vi "Humid Air Total Transfered Energy Calculator & OutPut Tempratures.vi"(2 "MFRHA\nMass Flow Rate of Humid Air (Kg/s)":dbl[unit], 3 "Gas Presure":dbl[unit]=80000.0 min=80000.0 max=120000.0, 4 "T_AU":dbl[unit], 5 "Tceg":dbl[unit], 6 "RH Heat Exchanger Quality":dbl, 7 "RH":dbl) -> (0 "Mass Flow Rate of Humid Air of Out Put":dbl[unit], 1 "ToTal Transferd Energy of Air":dbl[unit])   [LabVIEW 2018]
panel:
  out "T_AU\nEvaporator Hot and Humaid Outlet \nAir Temprature":dbl[unit](slide) scale=0.0..100.0
  out "ToTal Transferd Energy of Air":dbl[unit](slide) scale=0.0..5000.0
  out "Humidity of Input Air":dbl(knob) scale=0.0..100.0
  out "Temprature Of Input Air\nKelvin Degree":dbl[unit](slide) scale=273.0..373.0
  out "Tk":dbl[unit]
  out "Temprature Of Input Air\nCentigrade Degree":dbl[unit](slide) scale=0.0..100.0
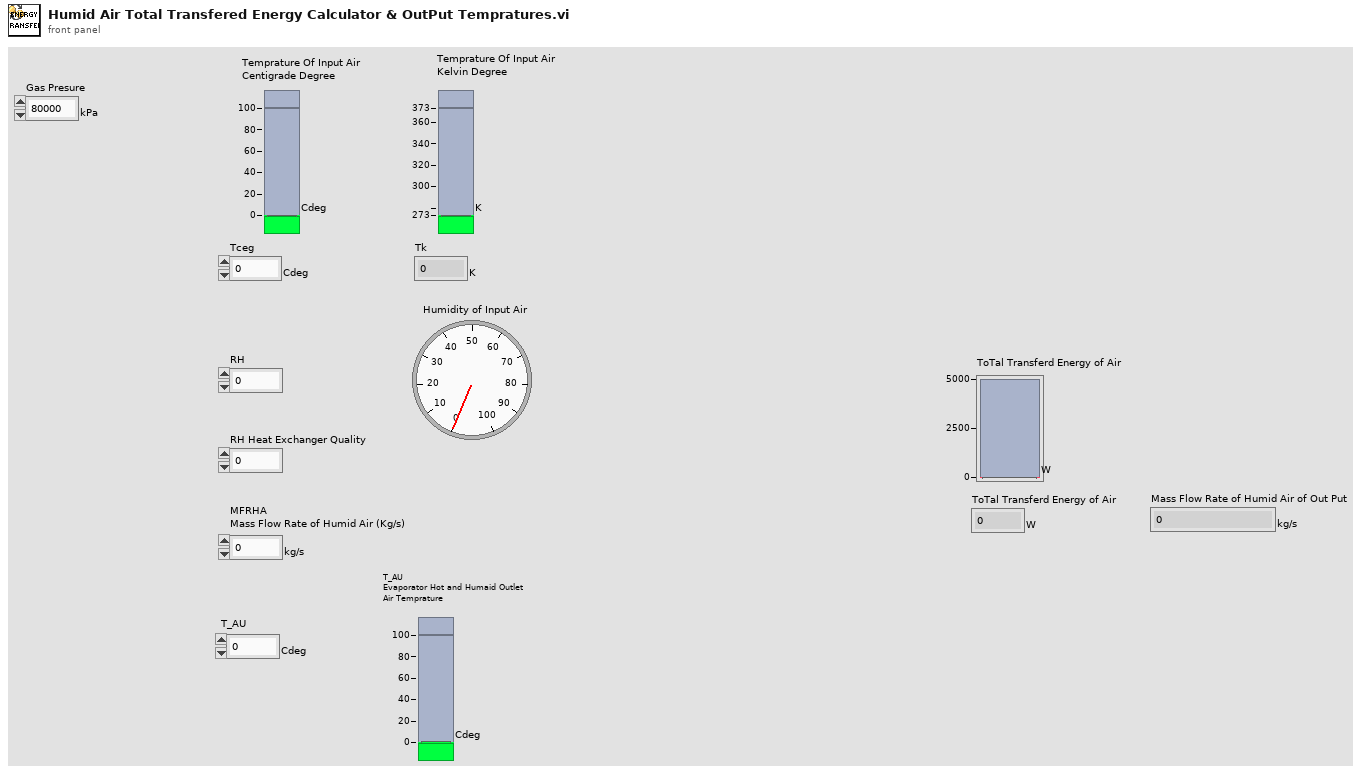
[diagram p1: front panel]
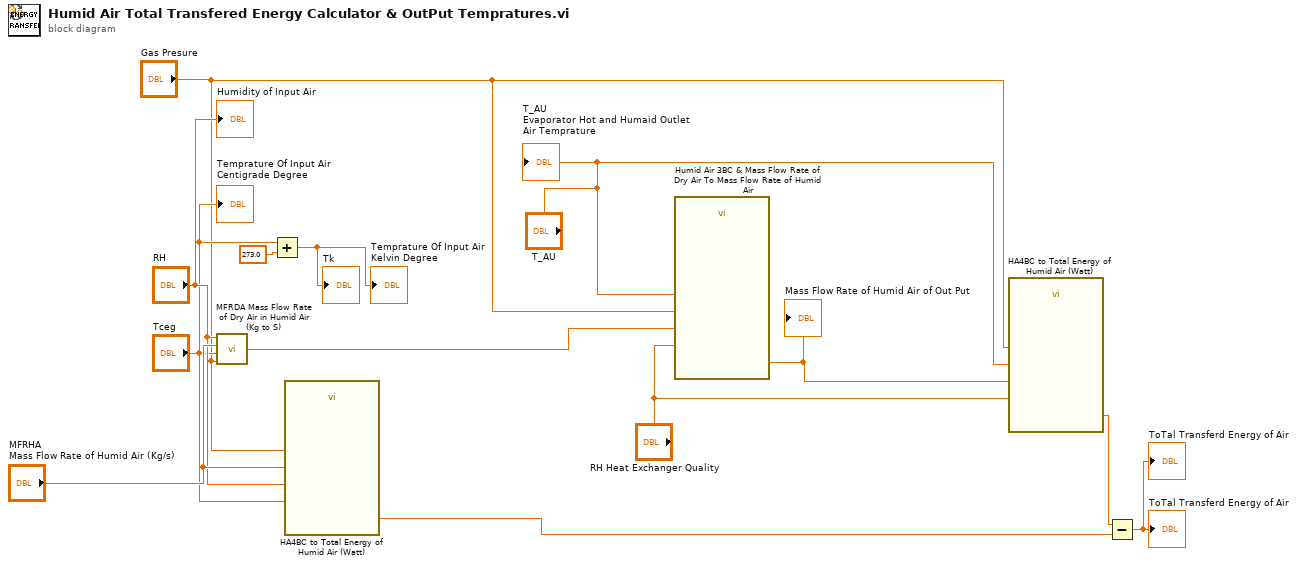
[diagram p0: block diagram]
diagram:
  n1 = call "MFRDA Mass Flow Rate of Dry Air in Humid Air (Kg to S).vi"("Gas Presure"="Gas Presure", "Tceg"="Tceg", "MFRHA\nMass Flow Rate of Humid Air (Kg/s)"="MFRHA\nMass Flow Rate of Humid Air (Kg/s)", "RH"="RH") -> ("MFRDA"=w11:dbl[unit])
  n2 = Add(x="Tceg", y=dbl[unit] 273.0) -> (x+y=→"Tk" →"Temprature Of Input Air\nKelvin Degree":dbl[unit])
  n3 = call "HA4BC to Total Energy of Humid Air (Watt).vi"("MFRHA\nMass Flow Rate of Humid Air (Kg/s)"="MFRHA\nMass Flow Rate of Humid Air (Kg/s)", "Gas Presure"="Gas Presure", "Tceg"="Tceg", "RH"="RH") -> ("Total Energy of Humid Air (Watt)"=w8:dbl[unit])
  n4 = call "Humid Air 3BC & Mass Flow Rate of Dry Air To Mass Flow Rate of Humid Air.vi"("Gas Presure"="Gas Presure", "Tceg"="T_AU", "M dot_DA"=w11, "RH"="RH Heat Exchanger Quality") -> ("Mdot_HA"=w6:dbl[unit])
  "Mass Flow Rate of Humid Air of Out Put" <- w6
  n5 = call "HA4BC to Total Energy of Humid Air (Watt).vi"("MFRHA\nMass Flow Rate of Humid Air (Kg/s)"=w6, "Gas Presure"="Gas Presure", "Tceg"="T_AU", "RH"="RH Heat Exchanger Quality") -> ("Total Energy of Humid Air (Watt)"=w7:dbl[unit])
  n6 = Subtract(x=w7, y=w8) -> (x-y=→"ToTal Transferd Energy of Air" →"ToTal Transferd Energy of Air":dbl[unit])
  "Temprature Of Input Air\nCentigrade Degree" <- "Tceg"
  "Humidity of Input Air" <- "RH"
  "T_AU\nEvaporator Hot and Humaid Outlet \nAir Temprature" <- "T_AU"
